vi "MARS_Flush_USB_Fifo.vi"(8 "error in (no error)":errorcluster, 11 "VISA Refnum in":refnum<visa-resource-name>) -> (0 "error out":errorcluster, 3 "VISA Refnum out":refnum<visa-resource-name>)   [LabVIEW 2015]
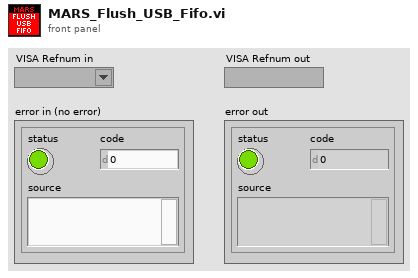
[diagram p1: front panel]
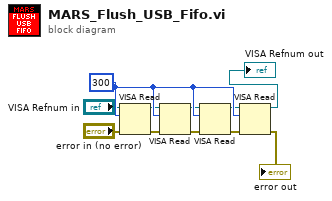
[diagram p0: block diagram]
diagram:
  w11 = u32 300 ("byte count")
  n1 = VISA Read(VISA resource name="VISA Refnum in", byte count=w11, error in (no error)="error in (no error)") -> (VISA resource name out=w3:refnum<visa-resource-name>, error out=w4:errorcluster)  [unwired: 2 out]
  n2 = VISA Read(VISA resource name=w3, byte count=w11, error in (no error)=w4) -> (VISA resource name out=w5:refnum<visa-resource-name>, error out=w6:errorcluster)  [unwired: 2 out]
  n3 = VISA Read(VISA resource name=w5, byte count=w11, error in (no error)=w6) -> (VISA resource name out=w7:refnum<visa-resource-name>, error out=w8:errorcluster)  [unwired: 2 out]
  n4 = VISA Read(VISA resource name=w7, byte count=w11, error in (no error)=w8) -> (VISA resource name out=→"VISA Refnum out":refnum<visa-resource-name>, error out=→"error out":errorcluster)  [unwired: 2 out]
